vi "Задание_АБ_рабочая_модуляция.vi"() -> ()   [LabVIEW 2017]
uses:
  <vilib>/Analysis/NI_AALBase.lvlib
panel:
  out "Модулирующий сигнал":dbl[](graph)
  out "Частотно модулированный цифровой сигнал":dbl[][](graph)
  in  "см. 1.2 Циклов в секунду":i32(slide) scale=4.0..50.0
  in  "Сколько битов брать":i32=4
  out "Радио сигнал с паузами":dbl[](graph)
  in  "Кол-во выборок":i32=400
  out "Массив с паузами":dbl[](array[numeric])
  in  "Количество бит":i32=8
  out "Вырезка из массива":dbl[](array[numeric])
  out "Биты на выходе 1":dbl[](array[numeric])
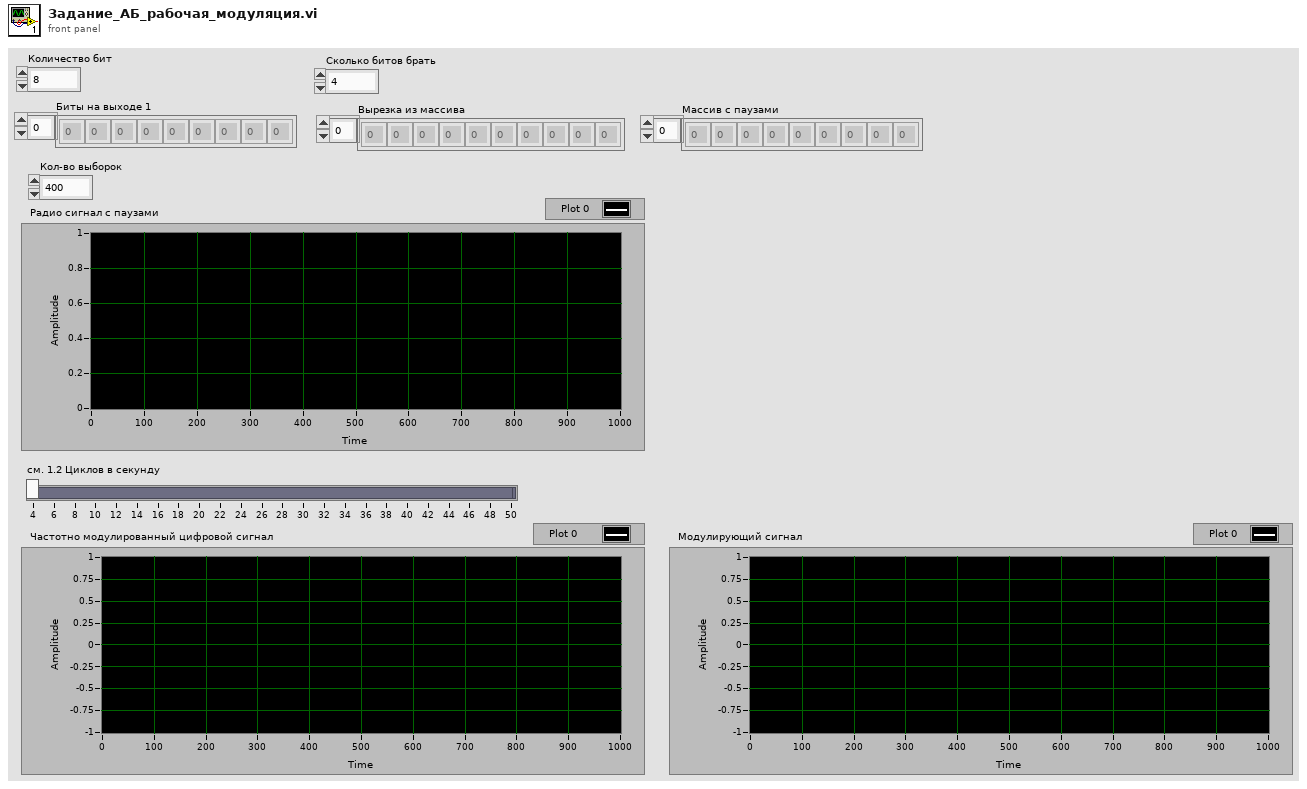
[diagram p1: front panel]
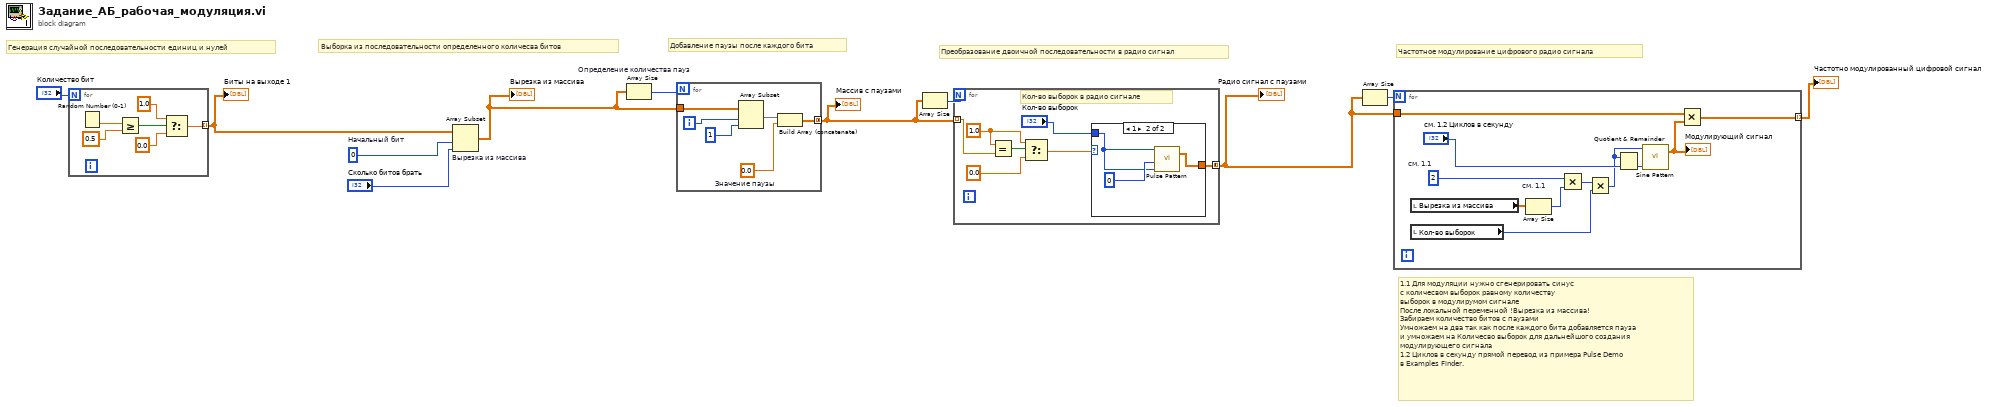
[diagram p0: block diagram]
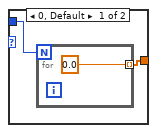
[diagram p2: hidden frame]
diagram:
  w10 = 0  # Начальный бит
  # "1.1 Для модуляции нужно сгенерировать синус \nс количесвом выборок равному количеству \nвыборок в модулирумом сигнале\nПосле локальной переменной !Вырезка из массива! \nЗабираем количество битов с паузами \nУмножаем на два так как после каждого бита добавляется пауза\nи умножаем на Количесво выборок для дальнейшого создания  \nмодулирующего сигнала\n1.2 Циклов в секунду прямой перевод из примера Pulse Demo \nв Examples Finder."
  # "Преобразование двоичной последовательности в радио сигнал"
  # "Частотное модулирование цифрового радио сигнала"
  # "Добавление паузы после каждого бита"
  # "Выборка из последовательности определенного количесва битов"
  # "Генерация случайной последовательности единиц и нулей"
  n1 = for {
    N: "Количество бит" -> [_]
    tunnel: [w12] -> w8 mode=indexing
    n2 = Random Number (0-1)() -> (number: 0 to 1=w17:dbl)
    n3 = Greater Or Equal?(x=w17, y=0.5) -> (x >= y?=w15:bool)
    n4 = Select(t=1.0, s=w15, f=0.0) -> (s? t:f=w12:dbl)
  }
  "Биты на выходе 1" <- w8
  n5 = Array Subset "Вырезка из массива"(array=w8, index=w10, length="Сколько битов брать") -> (w6:dbl[])
  "Вырезка из массива" <- w6
  n6 = Array Size "Определение количества пауз"(array=w6) -> (size(s)=w7:i32)
  n7 = for {
    N: w7 -> [_]
    tunnel: w6 -> [w20]
    tunnel: [w19] -> w3 mode=concatenating
    i -> [w18]
    w21 = 0.0  # Значение паузы
    n8 = Array Subset(array=w20, index=w18, length=1) -> (w22:dbl[])
    n9 = Build Array (concatenate)(w22, w21) -> (w19:dbl[])
  }
  "Массив с паузами" <- w3
  n10 = Array Size(array=w3) -> (size(s)=w4:i32)
  n11 = for {
    N: w4 -> [_]
    tunnel: w3 -> [w27] mode=indexing
    tunnel: [w25] -> w2 mode=concatenating
    w29 = 1.0
    # "Кол-во выборок в радио сигнале"
    n12 = Equal?(x=w29, y=w27) -> (x = y?=w30:bool)
    n13 = Select(t=w29, s=w30, f=0.0) -> (s? t:f=w26:dbl)
    n14 = case shown="1" w26 {
      tunnel: [w31 w35] -> w25
      tunnel: "Кол-во выборок" -> [w32 w34]
      frame 0, Default {
        n15 = for {
          N: w32 -> [_]
          tunnel: [0.0] -> w31 mode=indexing
        }
      }
      frame 1 {
        n16 = call <vilib>:"Pulse Pattern.vi"("width"=w34, "delay"=0, "samples"=w34) -> ("Pulse Pattern"=w35:dbl[])  [unwired: 1 in, 1 out]
      }
    }
  }
  "Радио сигнал с паузами" <- w2
  n17 = Array Size(array=w2) -> (size(s)=w5:i32)
  n18 = for {
    N: w5 -> [_]
    tunnel: w2 -> [w45]
    tunnel: [w44] -> w1 mode=indexing
    w40 = 2  # см. 1.1
    n19 = local read "Вырезка из массива"() -> (w42:dbl[])
    n20 = local read "Кол-во выборок"() -> (w38:i32)
    n21 = Array Size "см. 1.1"(array=w42) -> (size(s)=w41:i32)
    n22 = Multiply(x=w40, y=w41) -> (x*y=w39:i32)
    n23 = Multiply(x=w39, y=w38) -> (x*y=w37:i32)
    n24 = Quotient & Remainder(x=w37, y="см. 1.2 Циклов в секунду") -> (floor(x/y)=w47:i32)  [unwired: 1 out]
    n25 = call <vilib>:"Sine Pattern.vi"("cycles"=w47, "samples"=w37) -> ("Sinusoidal Pattern"=w43:dbl[])  [unwired: 2 in, 1 out]
    "Модулирующий сигнал" <- w43
    n26 = Multiply(x=w45, y=w43) -> (x*y=w44:dbl[])
  }
  "Частотно модулированный цифровой сигнал" <- w1
